vi "M1M3SupportEUI_View.vi"() -> ()   [LabVIEW 2016, in "M1M3SupportEUI_Views.lvlib"]
uses:
  M1M3SupportEUI_Views.lvlib
  Typedefs/StateTypes.ctl
  M1M3 Support Events/M1M3 Support Events.lvclass/M1M3 Support Events.ctl
  Warning Fault Tree View.vi
  Other Status.vi
  Inclinometer Graph View.vi
  Displacement Graph View.vi
  FA Values View.vi
  HP Values View.vi
  Typedefs/M1M3SupportEUI_TypeDefs.lvlib
  Controller/Controller.lvclass
  Settings/Settings.lvclass
  M1M3 Support Events/M1M3 Support Events.lvclass
  Model/Model.lvclass
panel:
  in  "Tab Control":T1(tab)
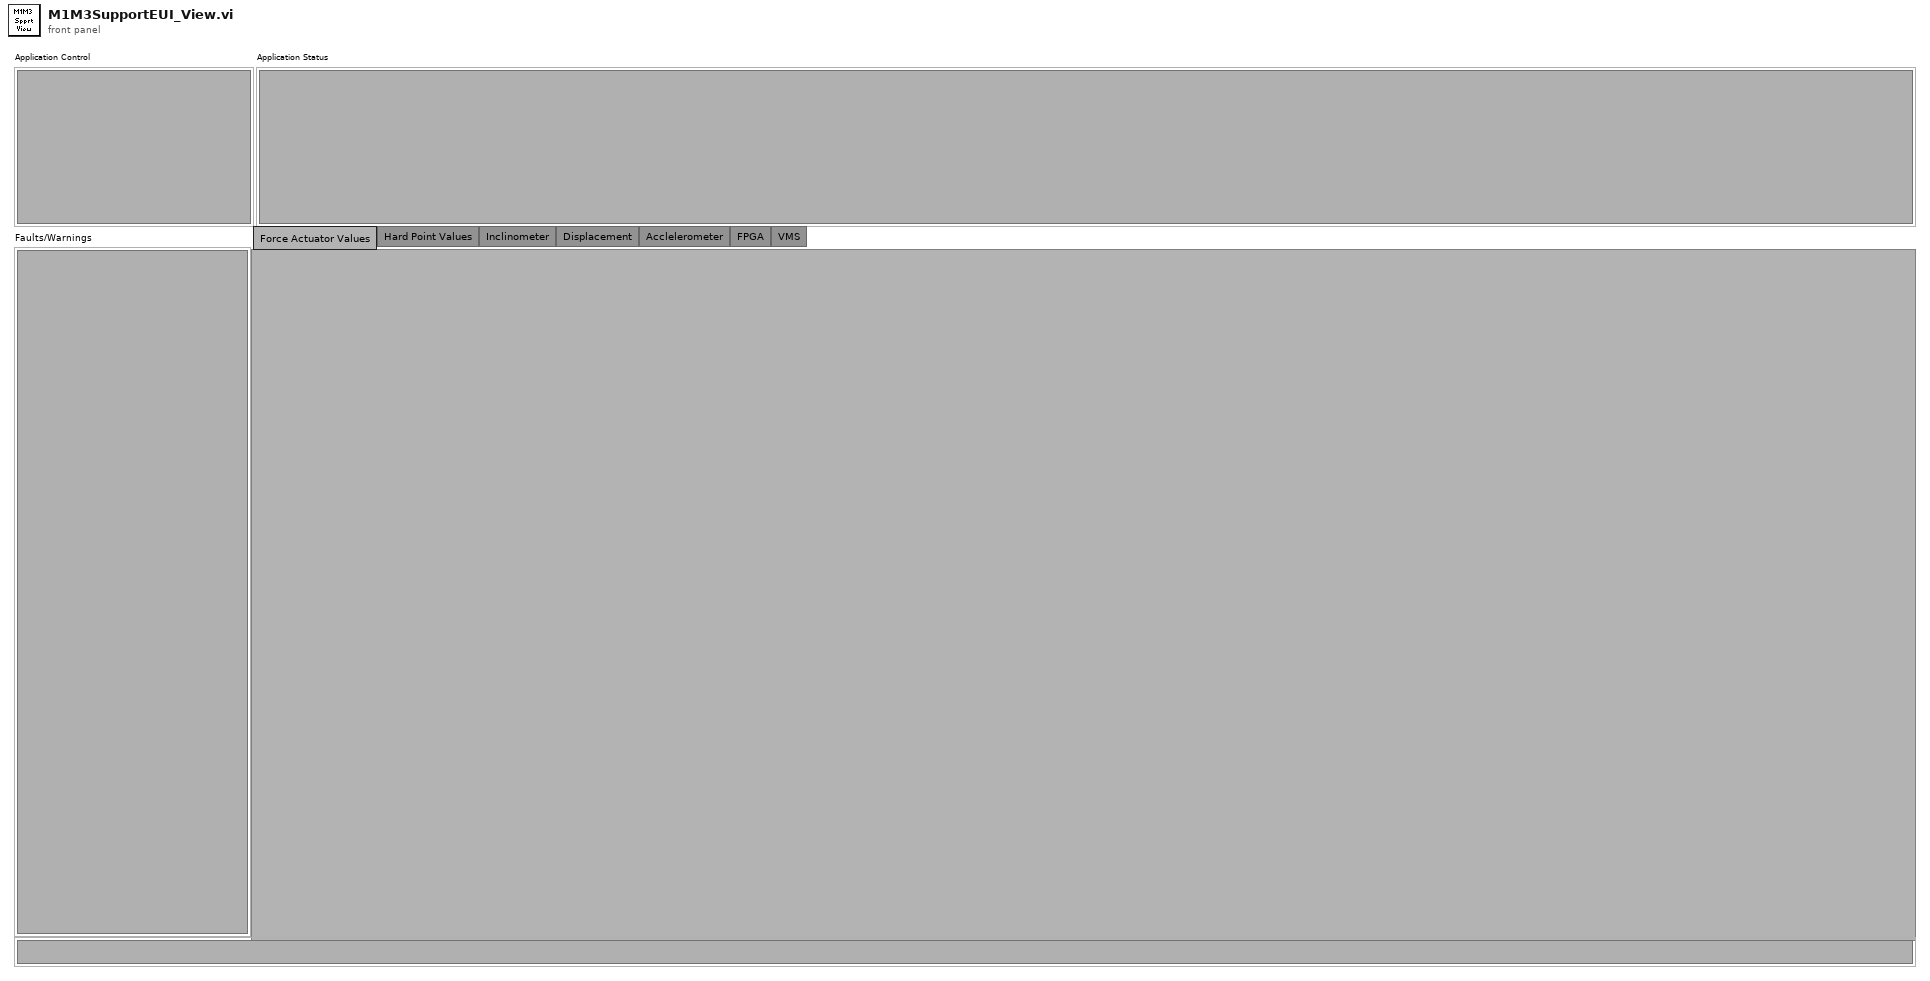
[diagram p1: front panel]
types:
  T1 = enum32{"Force Actuator Values", "Hard Point Values", "Inclinometer", "Displacement", "Acclelerometer", "FPGA", "VMS"}
  T2 = typedef "M1M3SupportEUI_TypeDefs.lvlib/StateTypes.ctl" = u32
  T3 = enum32{"invalid app kind", "Development System", "Run Time System", "Student Edition", "Embedded LabVIEW", "Evaluation", "Custom"}
  T4 = typedef "M1M3SupportEUI_TypeDefs.lvlib/M1M3 Support Events.ctl" = cluster{"M1M3 Support State":refnum<user-event>, "Inclinometer  Data":refnum<user-event>, "IMS Data":refnum<user-event>, "FA Data":refnum<user-event>, "FA Status":refnum<user-event>, "SAL Connected":refnum<user-event>, "HP Data":refnum<user-event>, "HP Status":refnum<user-event>}
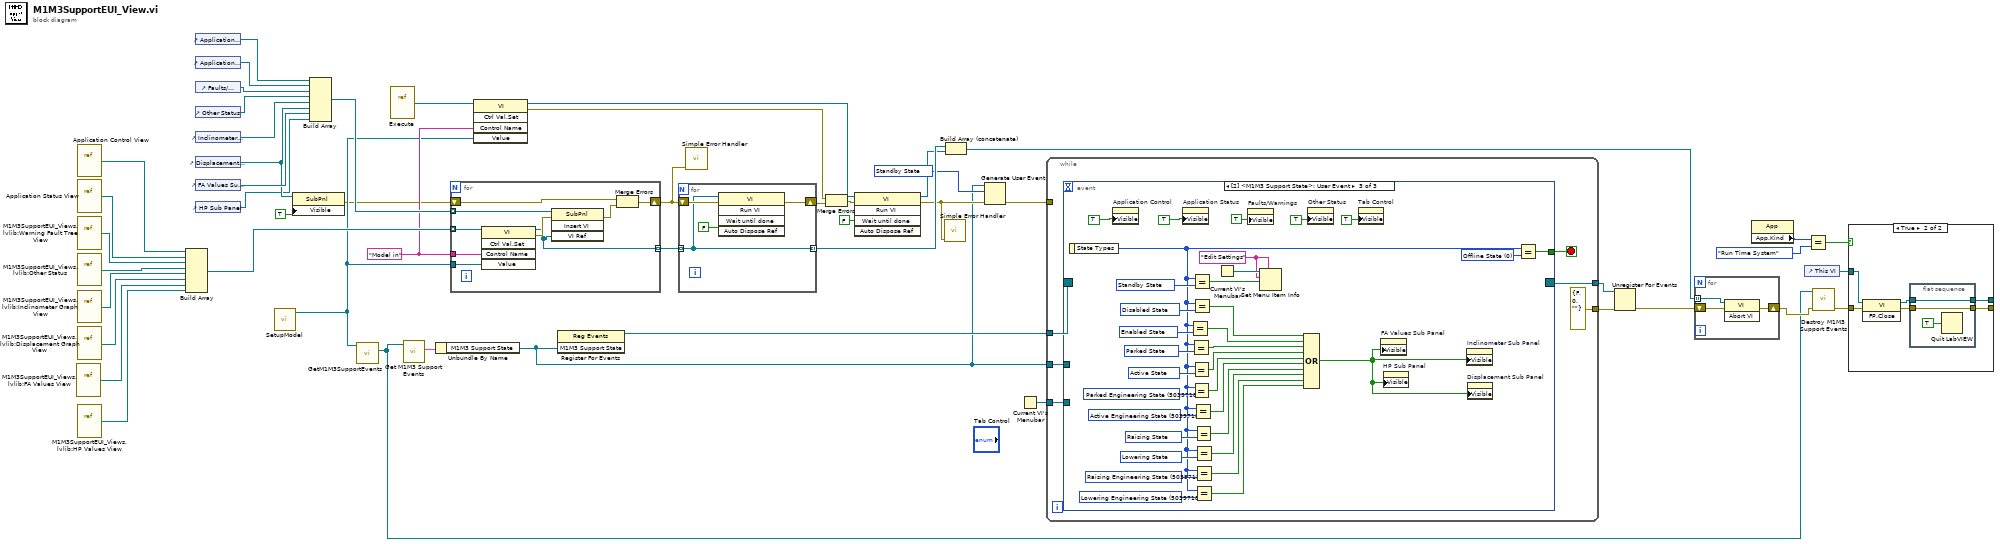
[diagram p0: block diagram]
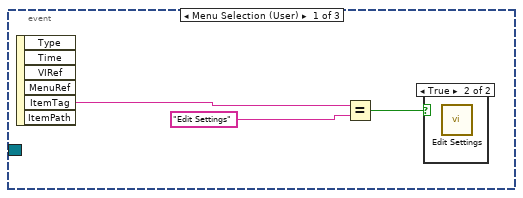
[diagram p2: hidden frame]
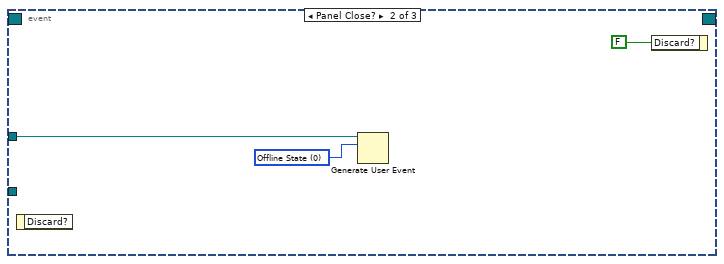
[diagram p4: hidden frame]
diagram:
  w16 = T2 16777216 items=["Offline State"=0, "Fault State"=4294967295, "Standby State"=16777216, "Disabled State"=33554432, "Enabled State"=50331648, "Parked State"=50331649, "Raising State"=50331650, "Active State"=50331651, "Lowering State"=50331652, "Engineering State"=50397184, "Parked Engineering State"=50397185, "Raising Engineering State"=50397186, "Active Engineering State"=50397187, "Lowering Engineering State"=50397188] ("event data")
  w23 = "Model in" ("Control Name")
  n1 = vi-ref "M1M3SupportEUI_Views.lvlib:FA Values View.vi"() -> (w9:refnum<vi>)
  n2 = vi-ref "Application Control View.vi"() -> (w2:refnum<vi>)
  n3 = vi-ref "Application Status View.vi"() -> (w34:refnum<vi>)
  n4 = vi-ref "M1M3SupportEUI_Views.lvlib:Warning Fault Tree View.vi"() -> (w28:refnum<vi>)
  n5 = vi-ref "M1M3SupportEUI_Views.lvlib:Other Status.vi"() -> (w26:refnum<vi>)
  n6 = vi-ref "M1M3SupportEUI_Views.lvlib:Inclinometer Graph View.vi"() -> (w25:refnum<vi>)
  n7 = vi-ref "M1M3SupportEUI_Views.lvlib:Displacement Graph View.vi"() -> (w24:refnum<vi>)
  n8 = vi-ref "M1M3SupportEUI_Views.lvlib:HP Values View.vi"() -> (w3:refnum<vi>)
  n9 = Build Array(w2, w34, w28, w26, w25, w24, w9, w3) -> (w33:refnum<vi>[])
  n10 = control-ref of="Application Control"() -> (w1:refnum<vi>)
  n11 = control-ref of="Application Status"() -> (w35:refnum<vi>)
  n12 = control-ref of="Faults/Warnings"() -> (w29:refnum<vi>)
  n13 = control-ref of="Other Status"() -> (w27:refnum<vi>)
  n14 = control-ref of="Inclinometer Sub Panel"() -> (w7:refnum<vi>)
  n15 = control-ref of="Displacement Sub Panel"() -> (w5:refnum<vi>)
  n16 = control-ref of="FA Values Sub Panel"() -> (w10:refnum<vi>)
  n17 = control-ref of="HP Sub Panel"() -> (w4:refnum<vi>)
  n18 = call "SetupModel.vi"() -> ("Model out"=w12:refnum<class "Model.lvclass">)  [unwired: 10 in, 1 out]
  n19 = property class="SubPnl"(reference=w5, "Visible"=TRUE) -> (error out=w6:errorcluster)  [unwired: 1 in, 1 out]
  n20 = Build Array(w1, w35, w29, w27, w7, w5, w10, w4) -> (w43:refnum<vi>[])
  n21 = call "GetM1M3SupportEvents.vi"("Model in"=w12) -> ("M1M3 Support Events out"=w11:refnum<class "M1M3 Support Events.lvclass">)  [unwired: 8 in, 2 out]
  n22 = vi-ref "Execute.vi"() -> (w32:refnum<vi>)
  n23 = call "Get M1M3 Support Events.vi"("M1M3 Support Events in"=w11) -> ("M1M3 Support Events"=w22:T4)  [unwired: 9 in, 1 out]
  n24 = Unbundle By Name(w22) -> ("M1M3 Support State"=w13:refnum<user-event>)
  n25 = for {
    tunnel: w43 -> [w59] mode=indexing
    tunnel: w33 -> [w51] mode=indexing
    shift-right: [w54] -> w36
    shift-left: w6 -> [w58]
    tunnel: [w55] -> w42 mode=indexing
    tunnel: w23 -> [w53]
    tunnel: w12 -> [w52]
    n26 = invoke class="VI" method="Ctrl Val.Set"(reference=w51, "Control Name"=w53, "Value"=w52) -> (reference out=w55:refnum<vi>, error out=w57:errorcluster)  [unwired: 2 in, 3 out]
    n27 = invoke on="Invoke Node" class="SubPnl" method="Insert VI"(reference=w59, error in=w57, "VI Ref"=w55) -> (error out=w56:errorcluster)  [unwired: 1 in, 3 out]
    n28 = Merge Errors(w58, w56) -> (w54:errorcluster)
  }
  n29 = invoke class="VI" method="Ctrl Val.Set"(reference=w32, "Control Name"=w23, "Value"=w12) -> (reference out=w31:refnum<vi>, error out=w30:errorcluster)  [unwired: 2 in, 3 out]
  n30 = register-events(w13) -> (reference out=w21:refnum<event-registration>)  [unwired: 2 in, 1 out]
  n31 = for {
    shift-right: [w63] -> w41
    shift-left: w36 -> [w62]
    tunnel: w42 -> [w60] mode=indexing
    tunnel: [w60] -> w39 mode=indexing
    n32 = invoke class="VI" method="Run VI"(reference=w60, error in=w62, "Wait until done"=FALSE ("Wait Until Done")) -> (error out=w63:errorcluster)  [unwired: 2 in, 4 out]
  }
  n33 = call <vilib>:"Simple Error Handler.vi"("error in (no error)"=w36) -> ()  [unwired: 4 in, 5 out]
  n34 = Merge Errors(w30, w41) -> (w40:errorcluster)
  n35 = invoke class="VI" method="Run VI"(reference=w31, error in=w40, "Wait until done"=FALSE ("Wait Until Done")) -> (reference out=w38:refnum<vi>, error out=w15:errorcluster)  [unwired: 2 in, 3 out]
  n36 = call <vilib>:"Simple Error Handler.vi"("error in (no error)"=w15) -> ()  [unwired: 4 in, 5 out]
  n37 = Build Array (concatenate)(w39, w38) -> (w37:refnum<vi>[])
  n38 = Generate User Event(user event=w13, event data cluster=w16, error in=w15) -> (error out=w14:errorcluster)  [unwired: 1 in, 1 out]
  n39 = Current VI's Menubar() -> (w46:refnum<k9>)
  n40 = while {
    tunnel: [errorcluster {"status"=FALSE, "code"=0, "source"=""} ("error out")] -> w45
    tunnel: w46 -> [w66]
    tunnel: w21 -> [w68]
    tunnel: [w65] -> w20
    tunnel: w14 -> [_]
    tunnel: w13 -> [w64]
    stop <- w67 stop-if-true
    n41 = event shown="[2] <M1M3 Support State>: User Event" {
      selector: w68 -> [_ _ _]
      dyn-events: [_ _ _] -> w65
      timeout: _ -> [_ _ _]
      tunnel: [_ _ w107] -> w67
      tunnel: w66 -> [_ _ _]
      tunnel: w64 -> [_ w74 _]
      event Menu Selection (User) {
        n42 = event-data() -> ("ItemTag"=w70:string)  [unwired: 1 in, 5 out]
        n43 = Equal?(x=w70, y="Edit Settings") -> (x = y?=w72:bool)
        n44 = case shown="True" w72 {
          frame False {
          }
          frame True {
            n45 = call "Edit Settings.vi"() -> ()  [unwired: 10 in, 2 out]
          }
        }
      }
      event Panel Close? {
        w73 = T2 0 items=["Offline State"=0, "Fault State"=4294967295, "Standby State"=16777216, "Disabled State"=33554432, "Enabled State"=50331648, "Parked State"=50331649, "Raising State"=50331650, "Active State"=50331651, "Lowering State"=50331652, "Engineering State"=50397184, "Parked Engineering State"=50397185, "Raising Engineering State"=50397186, "Active Engineering State"=50397187, "Lowering Engineering State"=50397188] ("event data")
        n46 = event-data() -> ()  [unwired: 1 in, 1 out]
        n47 = Generate User Event(user event=w74, event data cluster=w73) -> ()  [unwired: 2 in, 2 out]
        n48 = event-data("Discard?"=FALSE) -> ()  [unwired: 1 in, 1 out]
      }
      event User Event {
        w78 = T2 33554432 items=["Offline State"=0, "Fault State"=4294967295, "Standby State"=16777216, "Disabled State"=33554432, "Enabled State"=50331648, "Parked State"=50331649, "Raising State"=50331650, "Active State"=50331651, "Lowering State"=50331652, "Engineering State"=50397184, "Parked Engineering State"=50397185, "Raising Engineering State"=50397186, "Active Engineering State"=50397187, "Lowering Engineering State"=50397188] ("y")
        w84 = T2 50397188 items=["Offline State"=0, "Fault State"=4294967295, "Standby State"=16777216, "Disabled State"=33554432, "Enabled State"=50331648, "Parked State"=50331649, "Raising State"=50331650, "Active State"=50331651, "Lowering State"=50331652, "Engineering State"=50397184, "Parked Engineering State"=50397185, "Raising Engineering State"=50397186, "Active Engineering State"=50397187, "Lowering Engineering State"=50397188] ("y")
        w85 = T2 50397186 items=["Offline State"=0, "Fault State"=4294967295, "Standby State"=16777216, "Disabled State"=33554432, "Enabled State"=50331648, "Parked State"=50331649, "Raising State"=50331650, "Active State"=50331651, "Lowering State"=50331652, "Engineering State"=50397184, "Parked Engineering State"=50397185, "Raising Engineering State"=50397186, "Active Engineering State"=50397187, "Lowering Engineering State"=50397188] ("y")
        w86 = T2 50331652 items=["Offline State"=0, "Fault State"=4294967295, "Standby State"=16777216, "Disabled State"=33554432, "Enabled State"=50331648, "Parked State"=50331649, "Raising State"=50331650, "Active State"=50331651, "Lowering State"=50331652, "Engineering State"=50397184, "Parked Engineering State"=50397185, "Raising Engineering State"=50397186, "Active Engineering State"=50397187, "Lowering Engineering State"=50397188] ("y")
        w87 = T2 50331650 items=["Offline State"=0, "Fault State"=4294967295, "Standby State"=16777216, "Disabled State"=33554432, "Enabled State"=50331648, "Parked State"=50331649, "Raising State"=50331650, "Active State"=50331651, "Lowering State"=50331652, "Engineering State"=50397184, "Parked Engineering State"=50397185, "Raising Engineering State"=50397186, "Active Engineering State"=50397187, "Lowering Engineering State"=50397188] ("y")
        w93 = T2 50397187 items=["Offline State"=0, "Fault State"=4294967295, "Standby State"=16777216, "Disabled State"=33554432, "Enabled State"=50331648, "Parked State"=50331649, "Raising State"=50331650, "Active State"=50331651, "Lowering State"=50331652, "Engineering State"=50397184, "Parked Engineering State"=50397185, "Raising Engineering State"=50397186, "Active Engineering State"=50397187, "Lowering Engineering State"=50397188] ("y")
        w94 = T2 50397185 items=["Offline State"=0, "Fault State"=4294967295, "Standby State"=16777216, "Disabled State"=33554432, "Enabled State"=50331648, "Parked State"=50331649, "Raising State"=50331650, "Active State"=50331651, "Lowering State"=50331652, "Engineering State"=50397184, "Parked Engineering State"=50397185, "Raising Engineering State"=50397186, "Active Engineering State"=50397187, "Lowering Engineering State"=50397188] ("y")
        w95 = T2 50331651 items=["Offline State"=0, "Fault State"=4294967295, "Standby State"=16777216, "Disabled State"=33554432, "Enabled State"=50331648, "Parked State"=50331649, "Raising State"=50331650, "Active State"=50331651, "Lowering State"=50331652, "Engineering State"=50397184, "Parked Engineering State"=50397185, "Raising Engineering State"=50397186, "Active Engineering State"=50397187, "Lowering Engineering State"=50397188] ("y")
        w96 = T2 50331649 items=["Offline State"=0, "Fault State"=4294967295, "Standby State"=16777216, "Disabled State"=33554432, "Enabled State"=50331648, "Parked State"=50331649, "Raising State"=50331650, "Active State"=50331651, "Lowering State"=50331652, "Engineering State"=50397184, "Parked Engineering State"=50397185, "Raising Engineering State"=50397186, "Active Engineering State"=50397187, "Lowering Engineering State"=50397188] ("y")
        w97 = T2 50331648 items=["Offline State"=0, "Fault State"=4294967295, "Standby State"=16777216, "Disabled State"=33554432, "Enabled State"=50331648, "Parked State"=50331649, "Raising State"=50331650, "Active State"=50331651, "Lowering State"=50331652, "Engineering State"=50397184, "Parked Engineering State"=50397185, "Raising Engineering State"=50397186, "Active Engineering State"=50397187, "Lowering Engineering State"=50397188] ("y")
        w105 = T2 16777216 items=["Offline State"=0, "Fault State"=4294967295, "Standby State"=16777216, "Disabled State"=33554432, "Enabled State"=50331648, "Parked State"=50331649, "Raising State"=50331650, "Active State"=50331651, "Lowering State"=50331652, "Engineering State"=50397184, "Parked Engineering State"=50397185, "Raising Engineering State"=50397186, "Active Engineering State"=50397187, "Lowering Engineering State"=50397188] ("y")
        w102 = "Edit Settings" ("menu tag")
        w108 = T2 0 items=["Offline State"=0, "Fault State"=4294967295, "Standby State"=16777216, "Disabled State"=33554432, "Enabled State"=50331648, "Parked State"=50331649, "Raising State"=50331650, "Active State"=50331651, "Lowering State"=50331652, "Engineering State"=50397184, "Parked Engineering State"=50397185, "Raising Engineering State"=50397186, "Active Engineering State"=50397187, "Lowering Engineering State"=50397188] ("y")
        n49 = event-data() -> ("State Types"=w77:T2)  [unwired: 1 in]
        n50 = property on="Application Control" class="SubPnl"("Visible"=TRUE) -> ()  [unwired: 2 in, 2 out]
        n51 = property on="Application Status" class="SubPnl"("Visible"=TRUE) -> ()  [unwired: 2 in, 2 out]
        n52 = Equal?(x=w77, y=w97) -> (x = y?=w92:bool)
        n53 = Equal?(x=w77, y=w96) -> (x = y?=w91:bool)
        n54 = Equal?(x=w77, y=w95) -> (x = y?=w90:bool)
        n55 = Equal?(x=w77, y=w94) -> (x = y?=w89:bool)
        n56 = Equal?(x=w77, y=w105) -> (x = y?=w103:bool)
        n57 = Equal?(x=w77, y=w78) -> (x = y?=w76:bool)
        n58 = Equal?(x=w77, y=w93) -> (x = y?=w88:bool)
        n59 = Equal?(x=w77, y=w87) -> (x = y?=w83:bool)
        n60 = Equal?(x=w77, y=w86) -> (x = y?=w82:bool)
        n61 = Equal?(x=w77, y=w85) -> (x = y?=w81:bool)
        n62 = Equal?(x=w77, y=w84) -> (x = y?=w80:bool)
        n63 = Current VI's Menubar() -> (w104:refnum<k9>)
        n64 = property on="Faults/Warnings" class="SubPnl"("Visible"=TRUE) -> ()  [unwired: 2 in, 2 out]
        n65 = Set Menu Item Info(7:w102, 9:w103, 10:w102, 11:w104) -> ()  [unwired: 3 in, 2 out]
        n66 = Compound Arithmetic op=OR(w76, w92, w91, w90, w89, w88, w83, w82, w81, w80) -> (w79:bool)
        n67 = property on="Other Status" class="SubPnl"("Visible"=TRUE) -> ()  [unwired: 2 in, 2 out]
        n68 = property on="Tab Control" class="TabCtl (strict)"("Visible"=TRUE) -> ()  [unwired: 2 in, 2 out]
        n69 = property on="FA Values Sub Panel" class="SubPnl"("Visible"=w79) -> ()  [unwired: 2 in, 2 out]
        n70 = property on="HP Sub Panel" class="SubPnl"("Visible"=w79) -> ()  [unwired: 2 in, 2 out]
        n71 = property on="Inclinometer Sub Panel" class="SubPnl"("Visible"=w79) -> ()  [unwired: 2 in, 2 out]
        n72 = property on="Displacement Sub Panel" class="SubPnl"("Visible"=w79) -> ()  [unwired: 2 in, 2 out]
        n73 = Equal?(x=w77, y=w108) -> (x = y?=w107:bool)
      }
    }
  }
  n74 = Unregister For Events(event registration refnum=w20, error in=w45) -> (error out=w17:errorcluster)
  n75 = for {
    tunnel: w37 -> [w109] mode=indexing
    shift-right: [w110] -> w19
    shift-left: w17 -> [w111]
    n76 = invoke class="VI" method="Abort VI"(reference=w109, error in=w111) -> (error out=w110:errorcluster)  [unwired: 1 in, 2 out]
  }
  n77 = property class="App"() -> ("App.Kind"=w50:T3)  [unwired: 2 in, 2 out]
  n78 = control-ref of="This VI"() -> (w44:refnum<vi>)
  n79 = Equal?(x=w50, y=T3."Run Time System") -> (x = y?=w48:bool)
  n80 = call "Destroy M1M3 Support Events.vi"("error in (no error)"=w19, "M1M3 Support Events in"=w11) -> ("error out"=w18:errorcluster)  [unwired: 8 in, 1 out]
  n81 = case shown="True" w48 {
    tunnel: w44 -> [w113 w119]
    tunnel: w18 -> [w112 w118]
    tunnel: [w113 w116] -> _
    tunnel: [w112 w114] -> _
    frame False {
    }
    frame True {
      n82 = invoke class="VI" method="FP.Close"(reference=w119, error in=w118) -> (reference out=w115:refnum<vi>, error out=w117:errorcluster)  [unwired: 1 in, 1 out]
      n83 = flat-sequence {
        tunnel: w117 -> [w120]
        tunnel: [w121] -> w116
        tunnel: w115 -> [w121]
        tunnel: [w120] -> w114
        frame #0 {
          n84 = Quit LabVIEW(quit? (T)=TRUE) -> ()
        }
      }
    }
  }
